vi "Generate d(x,y,z).vi"(3 "Translation":cluster{"X":dbl, "Y":dbl, "Z":dbl} {"Z" format="%.2f"; "Y" format="%.2f"; "X" format="%.2f"}) -> (0 "Transformation matrix":T1)   [LabVIEW 2024]
uses:
  <vilib>/Analysis/Matrix/Datatypes/RealMatrix.ctl
  <vilib>/Analysis/Matrix/NI_Matrix.lvlib
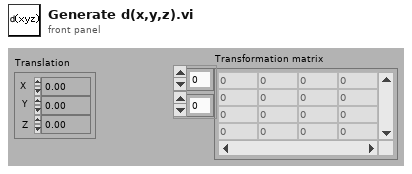
[diagram p1: front panel]
types:
  T1 = typedef "NI_Matrix.lvlib/RealMatrix.ctl" = dbl[][]
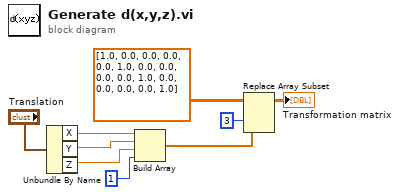
[diagram p0: block diagram]
diagram:
  n1 = Unbundle By Name("Translation") -> ("X"=w6:dbl, "Y"=w5:dbl, "Z"=w4:dbl)
  n2 = Build Array(w6, w5, w4, 1 ("Real Matrix Element")) -> (w2:dbl[])
  n3 = Replace Array Subset(array=dbl[][] [[1.0, 0.0, 0.0, 0.0], [0.0, 1.0, 0.0, 0.0], [0.0, 0.0, 1.0, 0.0], [0.0, 0.0, 0.0, 1.0]] ("Screw"), new element=w2, index (col)=3 ("disabled index (col)")) -> (→"Transformation matrix":dbl[][])  [unwired: 1 in]
